vi "target weighting.vi"(0 "Area":dbl, 2 "Width":dbl, 3 "Height":dbl, 4 "last offset":dbl, 5 "offset":dbl, 6 "bias":dbl) -> (7 "weighted offset":dbl)   [LabVIEW 2011]
panel:
  # "this VI will factor the robot's speed into how much we use the newest vision values (instead of factoring\nin previous iterations' more). Faster robot = more new data"
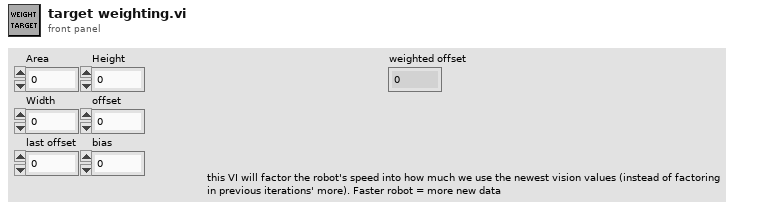
[diagram p1: front panel]
types:
  T1 = typedef "WPI_EncoderDevRef.ctl" = cluster{"DevStatus":errorcluster, "EncoderIndex":T2, "CounterIndex":T3, "DistancePerCount":dbl, "Decoding Type":T4}
  T2 = typedef "FPGA_EncoderIdx.ctl" = enum8{"Enc 0", "Enc 1", "Enc 2", "Enc 3", "Invalid"}
  T3 = typedef "FPGA_CounterCtrSystemIndex.ctl" = enum8{"Ctr 0", "Ctr 1", "Ctr 2", "Ctr 3", "Ctr 4", "Ctr 5", "Ctr 6", "Ctr 7", "Invalid"}
  T4 = typedef "WPI_EncoderType.ctl" = enum16{"1x", "2x", "4x"}
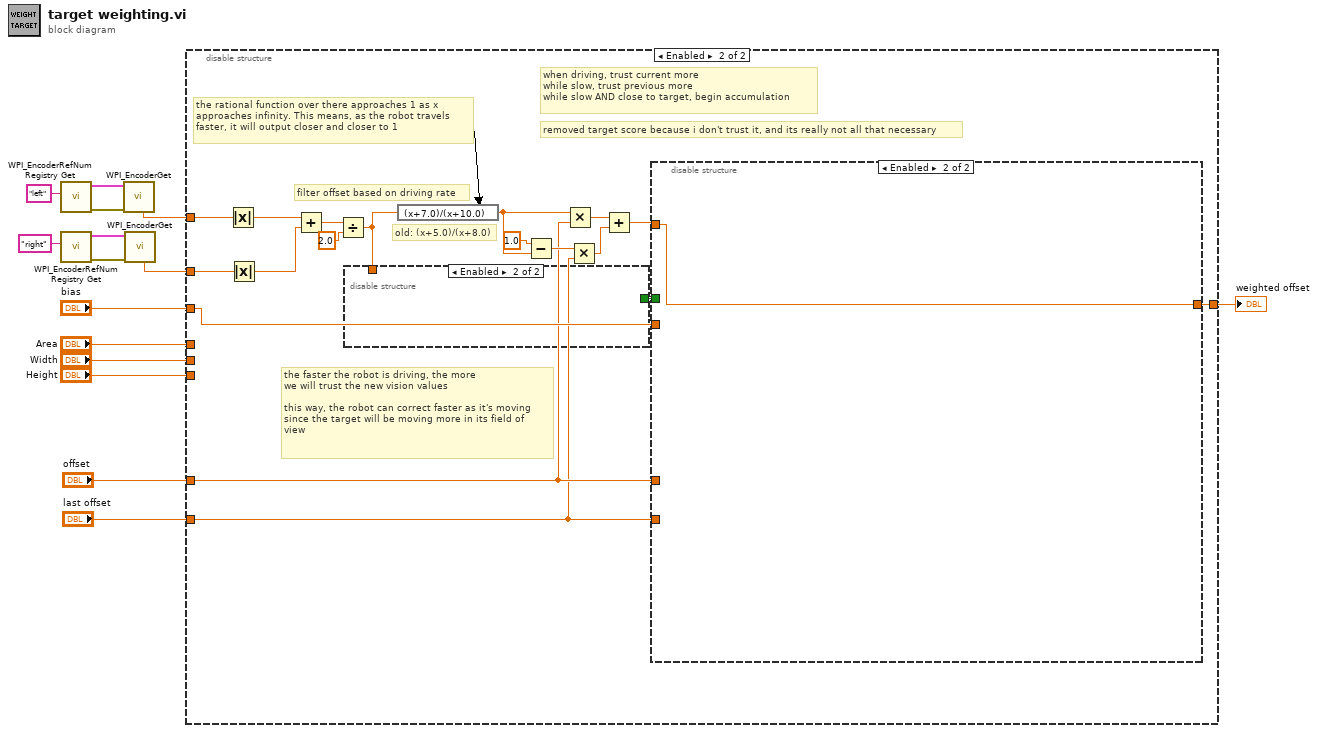
[diagram p0: block diagram]
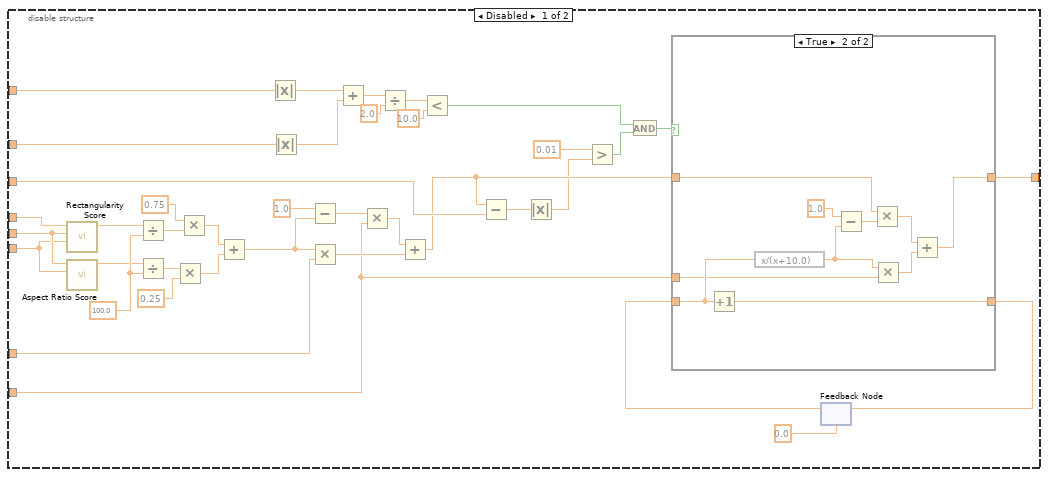
[diagram p2: hidden frame]
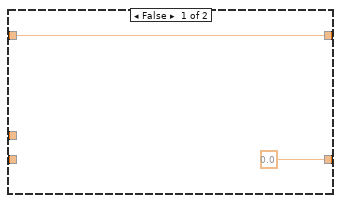
[diagram p3: hidden frame]
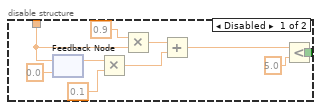
[diagram p4: hidden frame]
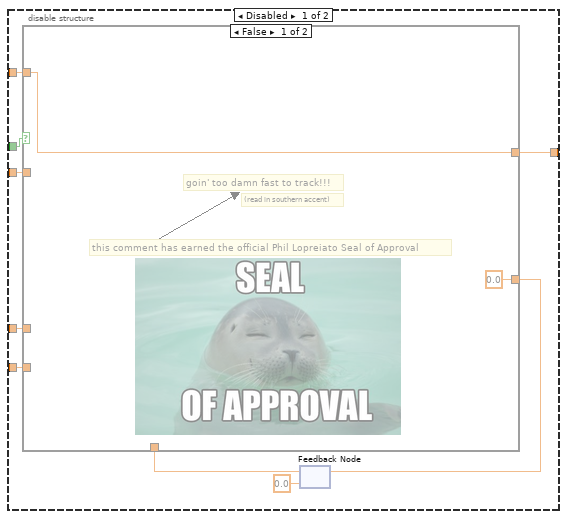
[diagram p5: hidden frame]
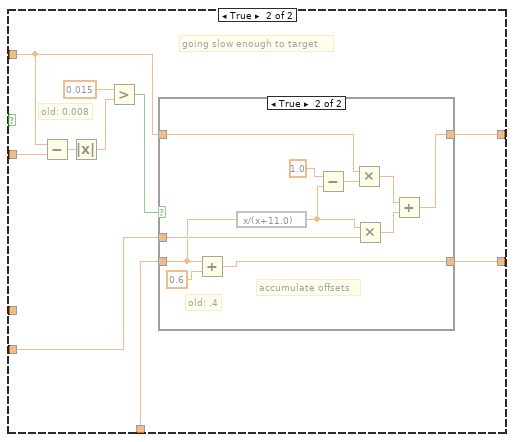
[diagram p6: hidden frame]
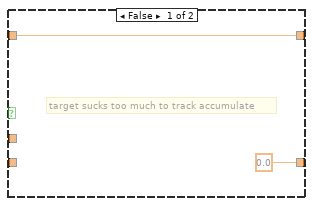
[diagram p7: hidden frame]
diagram:
  n1 = call <vilib>:"WPI_EncoderRefNum Registry Get.vi"("refnum name"="left") -> ("error out"=w7:errorcluster, "EncoderDevRef"=w9:T1)  [unwired: 9 in]
  n2 = call <vilib>:"WPI_EncoderRefNum Registry Get.vi"("refnum name"="right") -> ("error out"=w6:errorcluster, "EncoderDevRef"=w8:T1)  [unwired: 9 in]
  n3 = call <vilib>:"WPI_EncoderGet.vi"("error in (no error)"=w7, "EncoderDevRef"=w9) -> ("Rate"=w5:dbl)  [unwired: 4 in, 5 out]
  n4 = call <vilib>:"WPI_EncoderGet.vi"("error in (no error)"=w6, "EncoderDevRef"=w8) -> ("Rate"=w4:dbl)  [unwired: 4 in, 5 out]
  n5 = disable-structure shown="Enabled" {
    disable-tunnel: "Area" -> [w54 _]
    disable-tunnel: "Width" -> [w53 _]
    disable-tunnel: "Height" -> [w52 _]
    disable-tunnel: "offset" -> [w41 w70]
    disable-tunnel: w5 -> [w37 w80]
    disable-tunnel: w4 -> [w36 w79]
    disable-tunnel: [w28 w68] -> w3
    disable-tunnel: "last offset" -> [w27 w69]
    disable-tunnel: "bias" -> [w20 w71]
    frame Disabled {
      w50 = 100.0
      n6 = call "Rectangularity Score.vi"("Height"=w52, "Width"=w53, "Area"=w54) -> ("Score"=w51:dbl)  [unwired: 8 in]
      n7 = call "Aspect Ratio Score.vi"("Height"=w52, "Width"=w53) -> ("Score"=w49:dbl)  [unwired: 9 in]
      n8 = Divide(x=w51, y=w50) -> (x/y=w48:dbl)
      n9 = Divide(x=w49, y=w50) -> (x/y=w46:dbl)
      n10 = Multiply(x=w46, y=0.25) -> (x*y=w44:dbl)
      n11 = Multiply(x=0.75, y=w48) -> (x*y=w43:dbl)
      n12 = Add(x=w43, y=w44) -> (x+y=w26:dbl)
      n13 = Absolute Value(x=w37) -> (abs(x)=w22:dbl)
      n14 = Absolute Value(x=w36) -> (abs(x)=w21:dbl)
      n15 = Subtract(x=1.0, y=w26) -> (x-y=w40:dbl)
      n16 = Multiply(x=w26, y=w41) -> (x*y=w38:dbl)
      n17 = Add(x=w22, y=w21) -> (x+y=w35:dbl)
      n18 = Multiply(x=w40, y=w27) -> (x*y=w39:dbl)
      n19 = Divide(x=w35, y=2.0) -> (x/y=w33:dbl)
      n20 = Add(x=w39, y=w38) -> (x+y=w19:dbl)
      n21 = Less?(x=w33, y=10.0) -> (x < y?=w25:bool)
      n22 = Subtract(x=w19, y=w20) -> (x-y=w17:dbl)
      n23 = Absolute Value(x=w17) -> (abs(x)=w16:dbl)
      n24 = Greater?(x=0.01 ("y"), y=w16) -> (0:w24:bool)
      n25 = And(x=w25, y=w24) -> (x .and. y?=w23:bool)
      n26 = feedback #1(0.0) -> (w30:dbl)
      n27 = case shown="True" w23 {
        tunnel: w19 -> [w55 w62]
        tunnel: [0.0 ("Numeric") w65] -> w31
        tunnel: w30 -> [_ w66]
        tunnel: [w55 w57] -> w28
        tunnel: w27 -> [_ w61]
        frame False {
        }
        frame True {
          n28 = Increment(x=w66) -> (x+1=w65:dbl)
          n29 = expression code="x/(x+10.0)"(w66) -> (w60:dbl)
          n30 = Subtract(x=1.0, y=w60) -> (x-y=w63:dbl)
          n31 = Multiply(x=w62, y=w63) -> (x*y=w58:dbl)
          n32 = Multiply(x=w60, y=w61) -> (x*y=w59:dbl)
          n33 = Add(x=w58, y=w59) -> (x+y=w57:dbl)
        }
      }
      n34 = feedback-in #1(w31) -> ()
    }
    frame Enabled {
      # "the rational function over there approaches 1 as x \napproaches infinity. This means, as the robot travels \nfaster, it will output closer and closer to 1"
      # "the faster the robot is driving, the more\nwe will trust the new vision values\n\nthis way, the robot can correct faster as it's moving\nsince the target will be moving more in its field of\nview"
      # "old: (x+5.0)/(x+8.0)"
      # "removed target score because i don't trust it, and its really not all that necessary"
      # "when driving, trust current more\nwhile slow, trust previous more\nwhile slow AND close to target, begin accumulation"
      # "filter offset based on driving rate"
      n35 = Absolute Value(x=w80) -> (abs(x)=w83:dbl)
      n36 = Absolute Value(x=w79) -> (abs(x)=w84:dbl)
      n37 = Add(x=w83, y=w84) -> (x+y=w81:dbl)
      n38 = Divide(x=w81, y=2.0) -> (x/y=w67:dbl)
      n39 = disable-structure shown="Enabled" {
        disable-tunnel: [w93 _] -> w73
        disable-tunnel: w67 -> [w87 _]
        frame Disabled {
          n40 = feedback #2(0.0) -> (w91:dbl)
          n41 = feedback-in #2(w87) -> ()
          n42 = Multiply(x=w91, y=0.1) -> (x*y=w88:dbl)
          n43 = Multiply(x=0.9, y=w87) -> (x*y=w89:dbl)
          n44 = Add(x=w89, y=w88) -> (x+y=w85:dbl)
          n45 = Less?(x=w85, y=5.0) -> (x < y?=w93:bool)
        }
        frame Enabled {
        }
      }
      n46 = expression code="(x+7.0)/(x+10.0)"(w67) -> (w75:dbl)
      n47 = Subtract(x=1.0, y=w75) -> (x-y=w76:dbl)
      n48 = Multiply(x=w75, y=w70) -> (x*y=w78:dbl)
      n49 = Multiply(x=w76, y=w69) -> (x*y=w77:dbl)
      n50 = Add(x=w78, y=w77) -> (x+y=w72:dbl)
      n51 = disable-structure shown="Enabled" {
        disable-tunnel: w73 -> [w103 _]
        disable-tunnel: w72 -> [w102 w129]
        disable-tunnel: w71 -> [w101 _]
        disable-tunnel: w70 -> [w100 _]
        disable-tunnel: w69 -> [w99 _]
        disable-tunnel: [w98 w129] -> w68
        frame Disabled {
          n52 = feedback #3(0.0 ("Numeric")) -> (w95:dbl)
          n53 = case shown="False" w103 {
            tunnel: w102 -> [w105 w106]
            tunnel: w101 -> [_ w112]
            tunnel: w100 -> [_ _]
            tunnel: w99 -> [_ w110]
            tunnel: [w105 w109] -> w98
            tunnel: [0.0 ("Numeric") w108] -> w96
            tunnel: w95 -> [_ w107]
            frame False {
              # "this comment has earned the official Phil Lopreiato Seal of Approval"
              # "(read in southern accent)"
              # "goin' too damn fast to track!!!"
            }
            frame True {
              # "old: 0.008"
              # "going slow enough to target"
              n54 = Subtract(x=w106, y=w112) -> (x-y=w114:dbl)
              n55 = Absolute Value(x=w114) -> (abs(x)=w115:dbl)
              n56 = Greater?(x=0.015 ("y"), y=w115) -> (0:w111:bool)
              n57 = case shown="True" w111 {
                tunnel: w106 -> [w116 w126]
                tunnel: [0.0 ("Numeric") w120] -> w108
                tunnel: w107 -> [_ w119]
                tunnel: [w116 w121] -> w109
                tunnel: w110 -> [_ w125]
                frame False {
                  # "target sucks too much to track accumulate"
                }
                frame True {
                  # "old: .4"
                  # "accumulate offsets"
                  n58 = Add(x=w119, y=0.6) -> (x+y=w120:dbl)
                  n59 = expression code="x/(x+11.0)"(w119) -> (w124:dbl)
                  n60 = Subtract(x=1.0, y=w124) -> (x-y=w127:dbl)
                  n61 = Multiply(x=w126, y=w127) -> (x*y=w122:dbl)
                  n62 = Multiply(x=w124, y=w125) -> (x*y=w123:dbl)
                  n63 = Add(x=w122, y=w123) -> (x+y=w121:dbl)
                }
              }
            }
          }
          n64 = feedback-in #3(w96) -> ()
        }
        frame Enabled {
        }
      }
    }
  }
  "weighted offset" <- w3
